vi "Check_Fiber_Connection.vi"(8 "错误输入（无错误）":errorcluster, 9 "TSL":refnum<k24>[](array[refnum]), 10 "TSL_OSUport":dbl[](array[numeric]), 11 ".NET引用句柄输入":refnum<k24>) -> (0 "error out":errorcluster)   [LabVIEW 2017]
doc: "check fiber connection between TSL and OSU"
uses:
  LV_IL_Sample/DLL/InstrumentDLL.dll
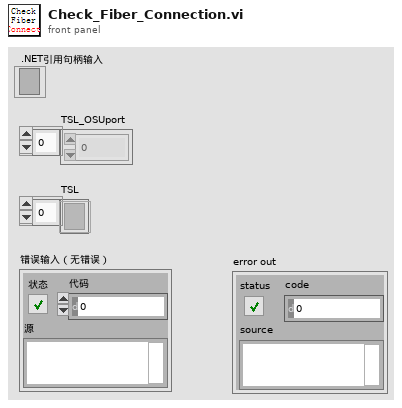
[diagram p1: front panel]
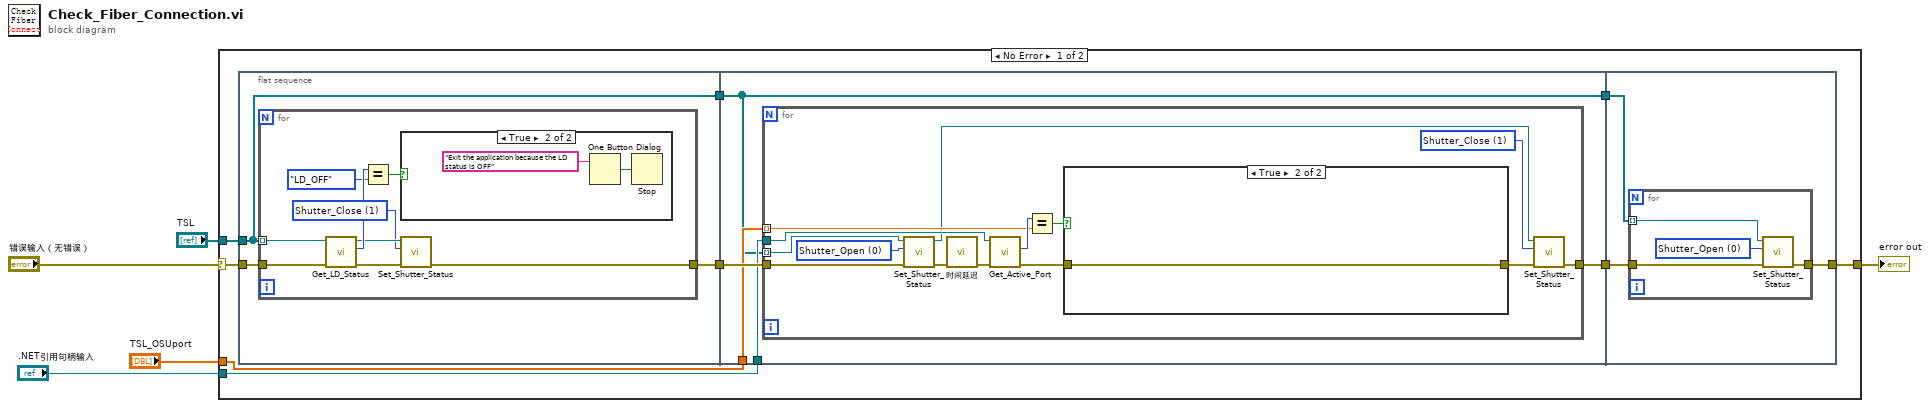
[diagram p0: block diagram]
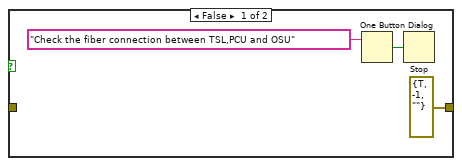
[diagram p3: hidden frame]
diagram:
  n1 = case shown="No Error" "错误输入（无错误）" {
    selector: "错误输入（无错误）" -> [w6 w59]
    tunnel: "TSL_OSUport" -> [w10 _]
    tunnel: ".NET引用句柄输入" -> [w9 _]
    tunnel: "TSL" -> [w8 _]
    tunnel: [w7 w59] -> w2
    frame No Error {
      n2 = flat-sequence {
        tunnel: w8 -> [w17]
        tunnel: [w17] -> w14
        tunnel: w6 -> [w16]
        tunnel: [w15] -> w13
        tunnel: w14 -> [w30]
        tunnel: w13 -> [w33]
        tunnel: w9 -> [w32]
        tunnel: w10 -> [w31]
        tunnel: [w30] -> w12
        tunnel: [w29] -> w11
        tunnel: w12 -> [w54]
        tunnel: w11 -> [w53]
        tunnel: [w52] -> w7
        frame #0 {
          n3 = for {
            tunnel: w17 -> [w26] mode=indexing
            tunnel: w16 -> [w22]
            tunnel: [w18] -> w15
            w19 = 1 items=["Shutter_Open", "Shutter_Close"] ("status")
            n4 = call "Get_LD_Status.vi"("error in (no error)"=w22, ".NET Reference in"=w26) -> ("error out"=w20:errorcluster, "status"=w25:enum16{"LD_OFF", "LD_ON", ""}, "Reference out"=w21:refnum<k24>)  [unwired: 7 in]
            n5 = Equal?(x=w25, y=enum16{"LD_OFF", "LD_ON", ""}."LD_OFF") -> (x = y?=w23:bool)
            n6 = case shown="True" w23 {
              frame False {
              }
              frame True {
                n7 = One Button Dialog(message="Exit the application because the LD status is OFF" ("消息")) -> (true=w27:bool)  [unwired: 1 in]
                n8 = Stop(stop? (T)=w27) -> ()
              }
            }
            n9 = call "Set_Shutter_Status.vi"(".NET Reference in"=w21, "status"=w19, "error in (no error)"=w20) -> ("error out"=w18:errorcluster)  [unwired: 6 in, 1 out]
          }
        }
        frame #1 {
          n10 = for {
            tunnel: w30 -> [w46] mode=indexing
            tunnel: w33 -> [w47]
            tunnel: w32 -> [w44]
            tunnel: w31 -> [w42] mode=indexing
            tunnel: [w36] -> w29
            w39 = 1 items=["Shutter_Open", "Shutter_Close"] ("status")
            w45 = 0 items=["Shutter_Open", "Shutter_Close"] ("status")
            n11 = call "Set_Shutter_Status.vi"(".NET Reference in"=w46, "status"=w45, "error in (no error)"=w47) -> ("Reference out"=w40:refnum<k24>, "error out"=w35:errorcluster)  [unwired: 6 in]
            n12 = call "时间延迟"("error in (no error)"=w35) -> ("error out"=w34:errorcluster)  [unwired: 10 in]
            n13 = call "Get_Active_Port.vi"("error in (no error)"=w34, ".NET Reference in"=w44) -> ("error out"=w37:errorcluster, "channel"=w43:u16)  [unwired: 7 in, 1 out]
            n14 = Equal?(x=w43, y=w42) -> (x = y?=w41:bool)
            n15 = case shown="True" w41 {
              tunnel: [errorcluster {"status"=TRUE, "code"=-1, "source"=""} ("错误常量") w51] -> w38
              tunnel: w37 -> [_ w51]
              frame False {
                n16 = One Button Dialog(message="Check the fiber connection between TSL,PCU and OSU" ("消息")) -> (true=w48:bool)  [unwired: 1 in]
                n17 = Stop(stop? (T)=w48) -> ()
              }
              frame True {
              }
            }
            n18 = call "Set_Shutter_Status.vi"(".NET Reference in"=w40, "status"=w39, "error in (no error)"=w38) -> ("error out"=w36:errorcluster)  [unwired: 6 in, 1 out]
          }
        }
        frame #2 {
          n19 = for {
            tunnel: w54 -> [w58] mode=indexing
            tunnel: w53 -> [w57]
            tunnel: [w55] -> w52
            w56 = 0 items=["Shutter_Open", "Shutter_Close"] ("status")
            n20 = call "Set_Shutter_Status.vi"(".NET Reference in"=w58, "status"=w56, "error in (no error)"=w57) -> ("error out"=w55:errorcluster)  [unwired: 6 in, 1 out]
          }
        }
      }
    }
    frame Error {
    }
  }
  "error out" <- w2
